vi "pc_write_control.vi"(0 "Write Previous":bool, 1 "Write Current":bool, 2 "Cont_info":string, 3 "Previous Data":string, 4 "Current Data":string, 5 "Frame Number":u32, 6 "Base Path":path, 7 "error in":errorcluster, 8 "mouseid":string, 10 "Box Number":u32) -> (19 "error out":errorcluster)   [LabVIEW 2013]
doc: "Build an appropriate path for writing data, then take current and/or previous data as strings and send them to be written."
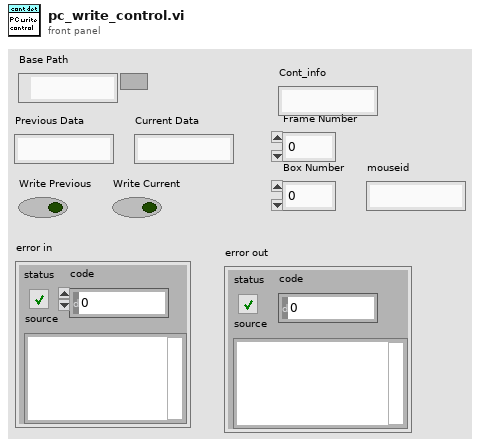
[diagram p1: front panel]
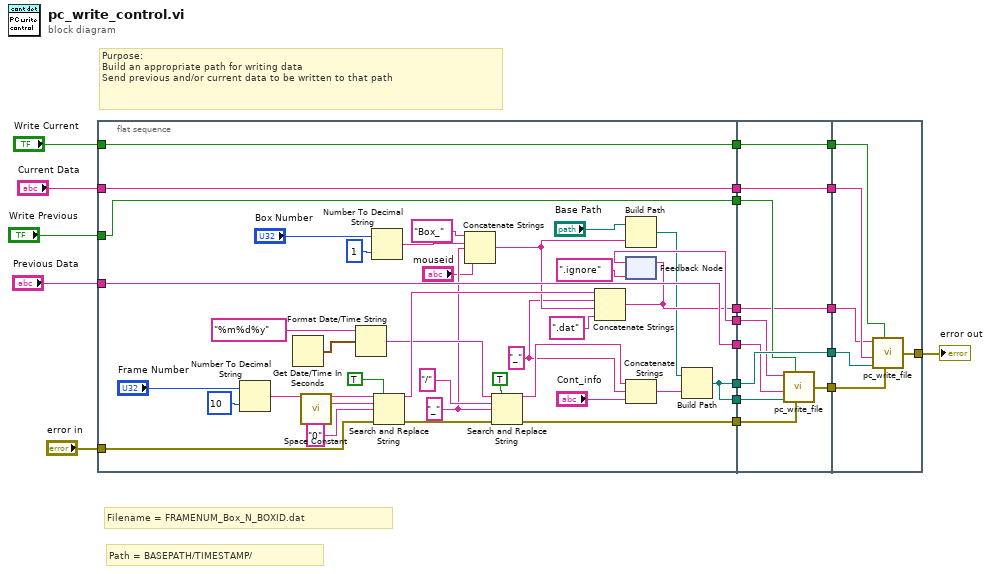
[diagram p0: block diagram]
diagram:
  # "Path = BASEPATH/TIMESTAMP/"
  # "Filename = FRAMENUM_Box_N_BOXID.dat"
  # "Purpose:\nBuild an appropriate path for writing data\nSend previous and/or current data to be written to that path"
  n1 = flat-sequence {
    tunnel: "Current Data" -> [w54]
    tunnel: "Previous Data" -> [w55]
    tunnel: "Write Current" -> [w56]
    tunnel: "Write Previous" -> [w57]
    tunnel: [w57] -> w20
    tunnel: [w56] -> w19
    tunnel: [w55] -> w18
    tunnel: [w54] -> w17
    tunnel: [w32] -> w16
    tunnel: [w32] -> w15
    tunnel: [w44] -> w14
    tunnel: "error in" -> [w36]
    tunnel: [w48] -> w3
    tunnel: [w50] -> w1
    tunnel: [w67] -> w13
    tunnel: w20 -> [w64]
    tunnel: w19 -> [w67]
    tunnel: w18 -> [w63]
    tunnel: w17 -> [w65]
    tunnel: w16 -> [w62]
    tunnel: [w66] -> w12
    tunnel: w15 -> [w66]
    tunnel: [w65] -> w11
    tunnel: w14 -> [w61]
    tunnel: [w60] -> w10
    tunnel: w3 -> [w58]
    tunnel: [w58] -> w2
    tunnel: w1 -> [w59]
    tunnel: w13 -> [w68]
    tunnel: w12 -> [w71]
    tunnel: w11 -> [w70]
    tunnel: w10 -> [w73]
    tunnel: [w72] -> w4
    tunnel: w2 -> [w69]
    frame #0 {
      w28 = "_"
      w22 = "_" ("replace string (\"\")")
      n2 = Number To Decimal String(number="Frame Number", width (-)=i16 10) -> (decimal integer string=w39:string)
      n3 = Get Date/Time In Seconds() -> (seconds since 1Jan1904=w26:timestamp)
      n4 = call <vilib>:"Space Constant.vi"() -> ("String"=w38:string)
      n5 = Format Date/Time String(time format string (%c)="%m%d%y", seconds (now)=w26) -> (date/time string=w24:string)  [unwired: 1 in]
      n6 = Number To Decimal String(number="Box Number", width (-)=i16 1) -> (decimal integer string=w47:string)
      n7 = Search and Replace String(replace all?=TRUE ("replace all? (F)"), input string=w39, search string=w38, replace string="0" ("replace string (\"\")"), error in=w36) -> (result string=w34:string, error out=w35:errorcluster)  [unwired: 3 in, 2 out]
      n8 = Concatenate Strings("Box_" ("string"), w47, w22, "mouseid") -> (w33:string)
      n9 = Search and Replace String(replace all?=TRUE ("replace all? (F)"), input string=w24, search string="/", replace string=w22, error in=w35) -> (result string=w30:string, error out=w44:errorcluster)  [unwired: 3 in, 2 out]
      n10 = Concatenate Strings(w34, w28, w33, ".dat" ("string")) -> (w48:string)
      n11 = Build Path(base path="Base Path", name or relative path=w33) -> (appended path=w31:path)
      n12 = feedback #1(".ignore") -> (w50:string)
      n13 = feedback-in #1(w48) -> ()
      n14 = Concatenate Strings(w30, w28, "Cont_info") -> (w27:string)
      n15 = Build Path(base path=w31, name or relative path=w27) -> (appended path=w32:path)
    }
    frame #1 {
      n16 = call "pc_write_file.vi"("error in"=w61, "Write Condition"=w64, "Base Path"=w62, "Data"=w63, "File Name"=w59) -> ("error out"=w60:errorcluster)  [unwired: 1 in]
    }
    frame #2 {
      n17 = call "pc_write_file.vi"("error in"=w73, "Write Condition"=w68, "Base Path"=w71, "Data"=w70, "File Name"=w69) -> ("error out"=w72:errorcluster)  [unwired: 1 in]
    }
  }
  "error out" <- w4
